vi "CRYDB Create Tables.vi"(8 "error in":errorcluster, 11 "connection reference":T1) -> (0 "error out":errorcluster, 3 "connection reference out":T1)   [LabVIEW 2013]
uses:
  <vilib>/addons/database/Connection.llb/Conn ObjectReference.ctl
  <vilib>/addons/database/Auxilliary.llb/DB Tools Column Info.ctl
  <vilib>/addons/database/Auxilliary.llb/DB Tools DataTypes.ctl
  <vilib>/addons/database/NI_Database_API.lvlib
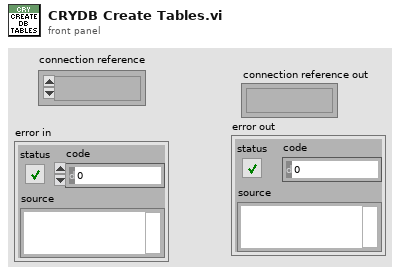
[diagram p1: front panel]
types:
  T1 = typedef "NI_Database_API.lvlib/Conn ObjectReference.ctl" = refnum<k1>
  T2 = typedef "NI_Database_API.lvlib/DB Tools Column Info.ctl" = cluster{"column name":string, "data type":T3, "size":i32, "allow null?":bool}
  T3 = typedef "NI_Database_API.lvlib/DB Tools DataTypes.ctl" = enum16{"String", "Long (I32)", "Single (SGL)", "Double (DBL)", "Date/Time", "Binary"}
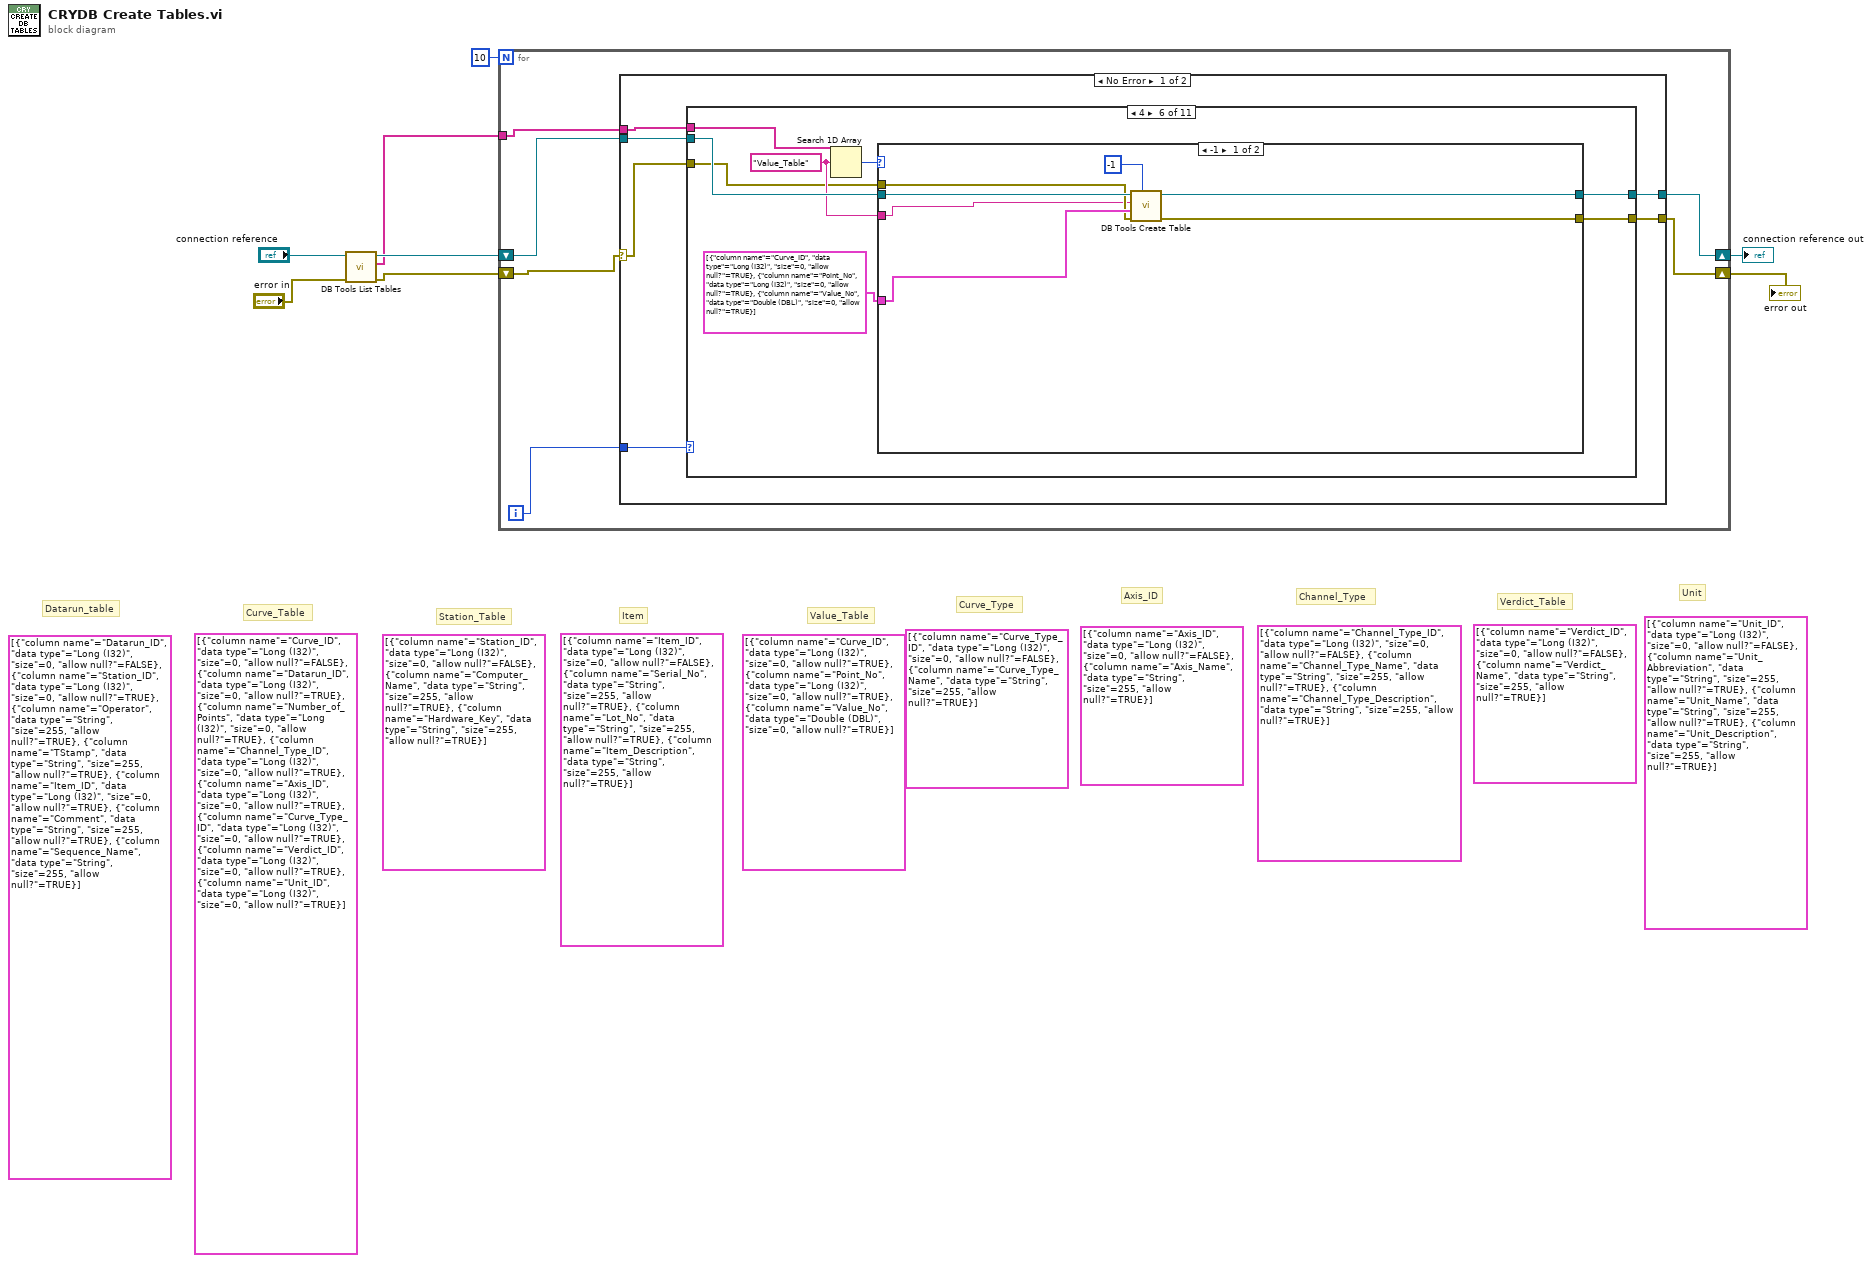
[diagram p0: block diagram]
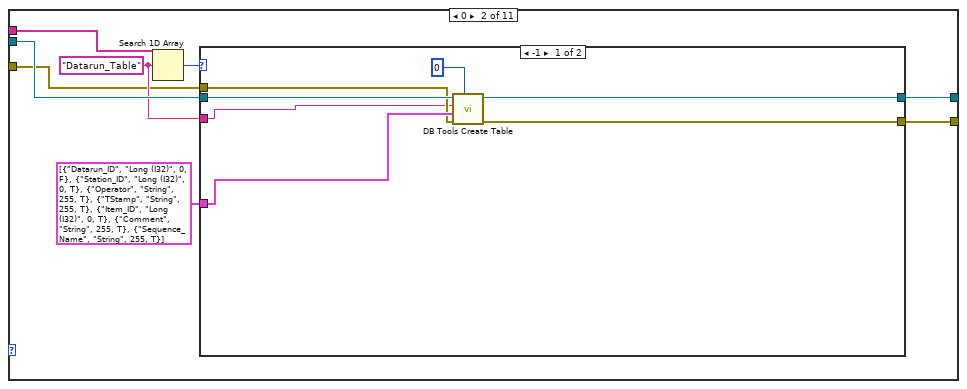
[diagram p3: hidden frame]
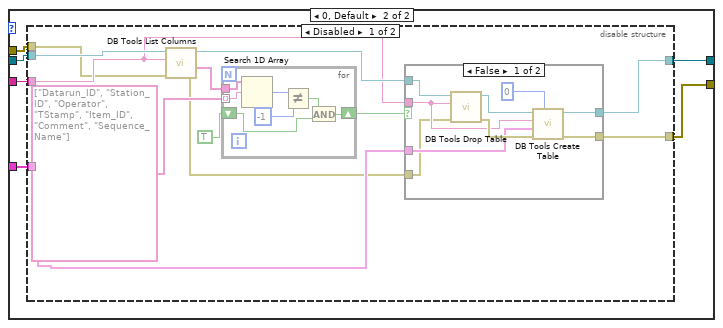
[diagram p4: hidden frame]
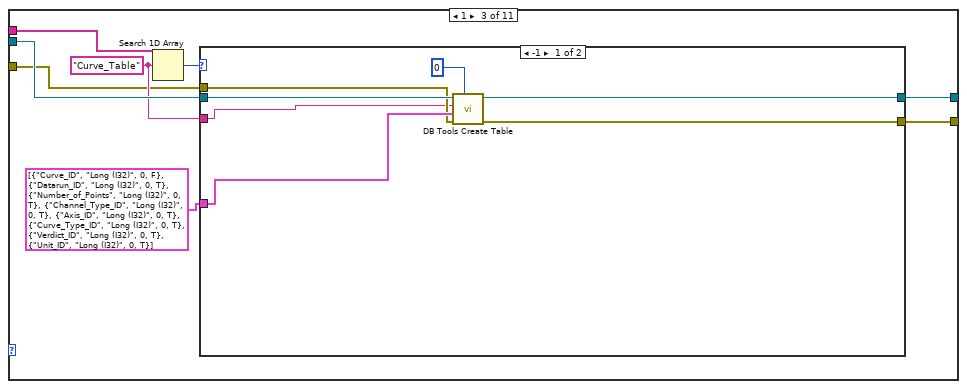
[diagram p7: hidden frame]
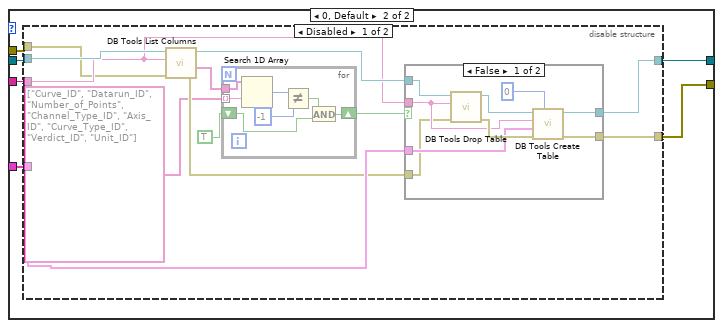
[diagram p8: hidden frame]
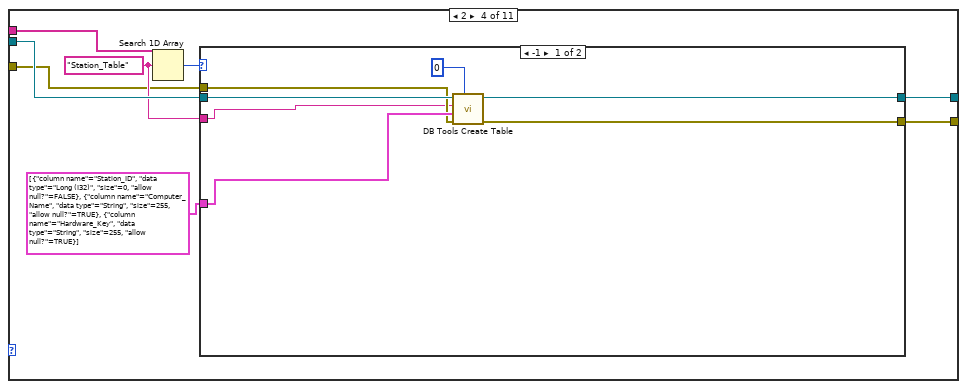
[diagram p11: hidden frame]
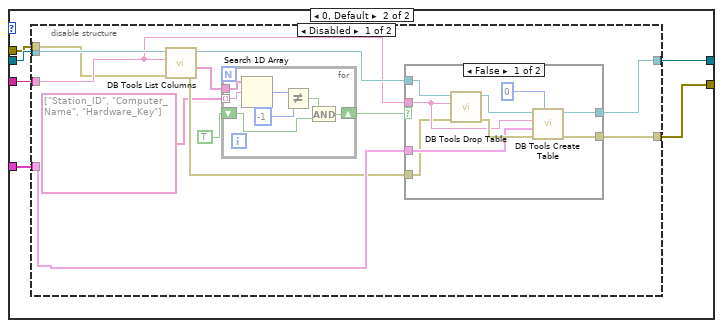
[diagram p12: hidden frame]
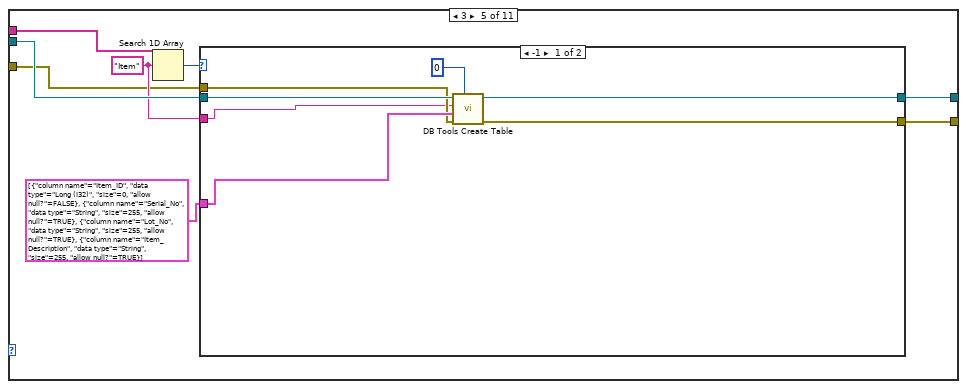
[diagram p15: hidden frame]
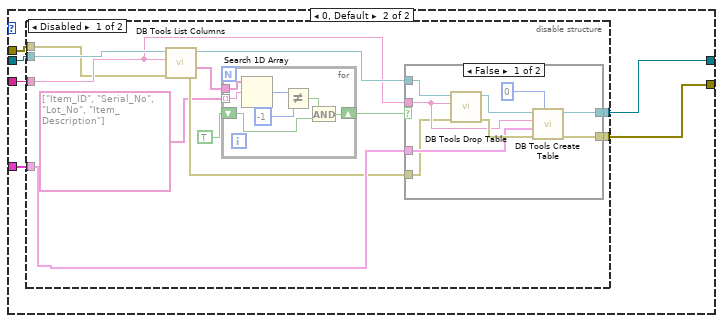
[diagram p16: hidden frame]
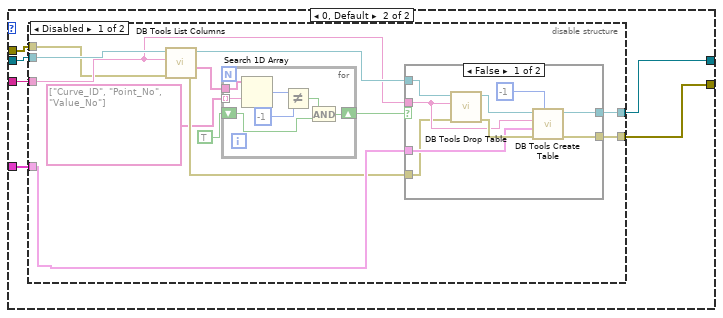
[diagram p19: hidden frame]
diagram:
  (unwired) T2[] [{"column name"="Unit_ID", "data type"=enum."Long (I32)", "size"=0, "allow null?"=FALSE}, {"column name"="Unit_Abbreviation", "data type"=enum."String", "size"=255, "allow null?"=TRUE}, {"column name"="Unit_Name", "data type"=enum."String", "size"=255, "allow null?"=TRUE}, {"column name"="Unit_Description", "data type"=enum."String", "size"=255, "allow null?"=TRUE}] ("column information")
  (unwired) T2[] [{"column name"="Verdict_ID", "data type"=enum."Long (I32)", "size"=0, "allow null?"=FALSE}, {"column name"="Verdict_Name", "data type"=enum."String", "size"=255, "allow null?"=TRUE}] ("column information")
  (unwired) T2[] [{"column name"="Channel_Type_ID", "data type"=enum."Long (I32)", "size"=0, "allow null?"=FALSE}, {"column name"="Channel_Type_Name", "data type"=enum."String", "size"=255, "allow null?"=TRUE}, {"column name"="Channel_Type_Description", "data type"=enum."String", "size"=255, "allow null?"=TRUE}] ("column information")
  (unwired) T2[] [{"column name"="Axis_ID", "data type"=enum."Long (I32)", "size"=0, "allow null?"=FALSE}, {"column name"="Axis_Name", "data type"=enum."String", "size"=255, "allow null?"=TRUE}] ("column information")
  (unwired) T2[] [{"column name"="Curve_Type_ID", "data type"=enum."Long (I32)", "size"=0, "allow null?"=FALSE}, {"column name"="Curve_Type_Name", "data type"=enum."String", "size"=255, "allow null?"=TRUE}] ("column information")
  (unwired) T2[] [{"column name"="Curve_ID", "data type"=enum."Long (I32)", "size"=0, "allow null?"=TRUE}, {"column name"="Point_No", "data type"=enum."Long (I32)", "size"=0, "allow null?"=TRUE}, {"column name"="Value_No", "data type"=enum."Double (DBL)", "size"=0, "allow null?"=TRUE}] ("column information")
  (unwired) T2[] [{"column name"="Item_ID", "data type"=enum."Long (I32)", "size"=0, "allow null?"=FALSE}, {"column name"="Serial_No", "data type"=enum."String", "size"=255, "allow null?"=TRUE}, {"column name"="Lot_No", "data type"=enum."String", "size"=255, "allow null?"=TRUE}, {"column name"="Item_Description", "data type"=enum."String", "size"=255, "allow null?"=TRUE}] ("column information")
  (unwired) T2[] [{"column name"="Station_ID", "data type"=enum."Long (I32)", "size"=0, "allow null?"=FALSE}, {"column name"="Computer_Name", "data type"=enum."String", "size"=255, "allow null?"=TRUE}, {"column name"="Hardware_Key", "data type"=enum."String", "size"=255, "allow null?"=TRUE}] ("column information")
  (unwired) T2[] [{"column name"="Curve_ID", "data type"=enum."Long (I32)", "size"=0, "allow null?"=FALSE}, {"column name"="Datarun_ID", "data type"=enum."Long (I32)", "size"=0, "allow null?"=TRUE}, {"column name"="Number_of_Points", "data type"=enum."Long (I32)", "size"=0, "allow null?"=TRUE}, {"column name"="Channel_Type_ID", "data type"=enum."Long (I32)", "size"=0, "allow null?"=TRUE}, {"column name"="Axis_ID", "data type"=enum."Long (I32)", "size"=0, "allow null?"=TRUE}, {"column name"="Curve_Type_ID", "data type"=enum."Long (I32)", "size"=0, "allow null?"=TRUE}, {"column name"="Verdict_ID", "data type"=enum."Long (I32)", "size"=0, "allow null?"=TRUE}, {"column name"="Unit_ID", "data type"=enum."Long (I32)", "size"=0, "allow null?"=TRUE}] ("column information")
  (unwired) T2[] [{"column name"="Datarun_ID", "data type"=enum."Long (I32)", "size"=0, "allow null?"=FALSE}, {"column name"="Station_ID", "data type"=enum."Long (I32)", "size"=0, "allow null?"=TRUE}, {"column name"="Operator", "data type"=enum."String", "size"=255, "allow null?"=TRUE}, {"column name"="TStamp", "data type"=enum."String", "size"=255, "allow null?"=TRUE}, {"column name"="Item_ID", "data type"=enum."Long (I32)", "size"=0, "allow null?"=TRUE}, {"column name"="Comment", "data type"=enum."String", "size"=255, "allow null?"=TRUE}, {"column name"="Sequence_Name", "data type"=enum."String", "size"=255, "allow null?"=TRUE}] ("column information")
  # "Unit"
  # "Verdict_Table"
  # "Channel_Type"
  # "Axis_ID"
  # "Curve_Type"
  # "Value_Table"
  # "Item"
  # "Station_Table"
  # "Curve_Table"
  # "Datarun_table"
  n1 = call <vilib>:"DB Tools List Tables.vi"("error in (no error)"="error in", "connection reference"="connection reference") -> ("error out"=w2:errorcluster, "tables"=w1:string[], "connection reference out"=w4:T1)  [unwired: 3 in]
  n2 = for {
    N: 10 -> [_]
    shift-right: [w12] -> w7
    shift-left: w4 -> [w14]
    shift-right: [w11] -> w6
    shift-left: w2 -> [w9]
    tunnel: w1 -> [w10]
    i -> [w13]
    n3 = case shown="No Error" w9 {
      selector: w9 -> [w15 w553]
      tunnel: w14 -> [w17 w554]
      tunnel: w13 -> [w20 _]
      tunnel: [w19 w554] -> w12
      tunnel: [w18 w553] -> w11
      tunnel: w10 -> [w16 _]
      frame No Error {
        n4 = case shown="4" w20 {
          tunnel: w16 -> [_ w30 w83 w136 w189 w242 w295 w348 w401 w454 w507]
          tunnel: w17 -> [w22 w29 w82 w135 w188 w241 w294 w347 w400 w453 w506]
          tunnel: [w22 w25 w79 w132 w185 w238 w291 w344 w397 w450 w503] -> w19
          tunnel: [w21 w24 w78 w131 w184 w237 w290 w343 w396 w449 w502] -> w18
          tunnel: w15 -> [w21 w23 w77 w130 w183 w236 w289 w342 w395 w448 w501]
          frame Default {
          }
          frame 0 {
            w27 = "Datarun_Table" ("element")
            n5 = Search 1D Array(1D array=w30, element=w27) -> (index of element=w28:i32)  [unwired: 1 in]
            n6 = case shown="-1" w28 {
              tunnel: w29 -> [w37 w43]
              tunnel: [w35 w40] -> w24
              tunnel: w27 -> [w31 w42]
              tunnel: T2[] [{"column name"="Datarun_ID", "data type"=enum."Long (I32)", "size"=0, "allow null?"=FALSE}, {"column name"="Station_ID", "data type"=enum."Long (I32)", "size"=0, "allow null?"=TRUE}, {"column name"="Operator", "data type"=enum."String", "size"=255, "allow null?"=TRUE}, {"column name"="TStamp", "data type"=enum."String", "size"=255, "allow null?"=TRUE}, {"column name"="Item_ID", "data type"=enum."Long (I32)", "size"=0, "allow null?"=TRUE}, {"column name"="Comment", "data type"=enum."String", "size"=255, "allow null?"=TRUE}, {"column name"="Sequence_Name", "data type"=enum."String", "size"=255, "allow null?"=TRUE}] ("column information") -> [w34 w41]
              tunnel: [w33 w39] -> w25
              tunnel: w23 -> [w32 w38]
              frame -1 {
                n7 = call <vilib>:"DB Tools Create Table.vi"("primary key (-1)"=0, "error in (no error)"=w32, "column information"=w34, "table"=w31, "connection reference"=w37) -> ("error out"=w35:errorcluster, "connection reference out"=w33:T1)  [unwired: 3 in]
              }
              frame 0, Default {
                n8 = disable-structure shown="Disabled" {
                  disable-tunnel: w43 -> [w55 w74]
                  disable-tunnel: w42 -> [w49 _]
                  disable-tunnel: w41 -> [w48 _]
                  disable-tunnel: [w47 w75] -> w40
                  disable-tunnel: [w46 w74] -> w39
                  disable-tunnel: w38 -> [w45 w75]
                  frame Disabled {
                    n9 = call <vilib>:"DB Tools List Columns.vi"("error in (no error)"=w45, "table"=w49, "connection reference"=w55) -> ("error out"=w44:errorcluster, "columns"=w53:string[], "connection reference out"=w50:T1)  [unwired: 1 in, 1 out]
                    n10 = for {
                      tunnel: string[] ["Datarun_ID", "Station_ID", "Operator", "TStamp", "Item_ID", "Comment", "Sequence_Name"] ("columns") -> [w72] mode=indexing
                      tunnel: w53 -> [w73]
                      shift-right: [w67] -> w51
                      shift-left: TRUE -> [w69]
                      n11 = Search 1D Array(1D array=w73, element=w72) -> (index of element=w71:i32)  [unwired: 1 in]
                      n12 = Not Equal?(x=w71, y=-1) -> (x != y?=w68:bool)
                      n13 = And(x=w68, y=w69) -> (x .and. y?=w67:bool)
                    }
                    n14 = case shown="False" w51 {
                      tunnel: w50 -> [w64 w66]
                      tunnel: w49 -> [w60 _]
                      tunnel: w48 -> [w61 _]
                      tunnel: [w58 w65] -> w47
                      tunnel: [w57 w66] -> w46
                      tunnel: w44 -> [w56 w65]
                      frame False {
                        n15 = call <vilib>:"DB Tools Drop Table.vi"("error in (no error)"=w56, "table"=w60, "connection reference"=w64) -> ("error out"=w62:errorcluster, "connection reference out"=w63:T1)  [unwired: 5 in]
                        n16 = call <vilib>:"DB Tools Create Table.vi"("primary key (-1)"=0, "error in (no error)"=w62, "column information"=w61, "table"=w60, "connection reference"=w63) -> ("error out"=w58:errorcluster, "connection reference out"=w57:T1)  [unwired: 3 in]
                      }
                      frame True {
                      }
                    }
                  }
                  frame Enabled {
                  }
                }
              }
            }
          }
          frame 1 {
            w80 = "Curve_Table" ("element")
            n17 = Search 1D Array(1D array=w83, element=w80) -> (index of element=w81:i32)  [unwired: 1 in]
            n18 = case shown="-1" w81 {
              tunnel: w82 -> [w90 w96]
              tunnel: [w88 w93] -> w78
              tunnel: w80 -> [w84 w95]
              tunnel: T2[] [{"column name"="Curve_ID", "data type"=enum."Long (I32)", "size"=0, "allow null?"=FALSE}, {"column name"="Datarun_ID", "data type"=enum."Long (I32)", "size"=0, "allow null?"=TRUE}, {"column name"="Number_of_Points", "data type"=enum."Long (I32)", "size"=0, "allow null?"=TRUE}, {"column name"="Channel_Type_ID", "data type"=enum."Long (I32)", "size"=0, "allow null?"=TRUE}, {"column name"="Axis_ID", "data type"=enum."Long (I32)", "size"=0, "allow null?"=TRUE}, {"column name"="Curve_Type_ID", "data type"=enum."Long (I32)", "size"=0, "allow null?"=TRUE}, {"column name"="Verdict_ID", "data type"=enum."Long (I32)", "size"=0, "allow null?"=TRUE}, {"column name"="Unit_ID", "data type"=enum."Long (I32)", "size"=0, "allow null?"=TRUE}] ("column information") -> [w87 w94]
              tunnel: [w86 w92] -> w79
              tunnel: w77 -> [w85 w91]
              frame -1 {
                n19 = call <vilib>:"DB Tools Create Table.vi"("primary key (-1)"=0, "error in (no error)"=w85, "column information"=w87, "table"=w84, "connection reference"=w90) -> ("error out"=w88:errorcluster, "connection reference out"=w86:T1)  [unwired: 3 in]
              }
              frame 0, Default {
                n20 = disable-structure shown="Disabled" {
                  disable-tunnel: w96 -> [w108 w128]
                  disable-tunnel: w95 -> [w103 _]
                  disable-tunnel: w94 -> [w102 _]
                  disable-tunnel: [w101 w127] -> w93
                  disable-tunnel: [w100 w128] -> w92
                  disable-tunnel: w91 -> [w99 w127]
                  frame Disabled {
                    n21 = call <vilib>:"DB Tools List Columns.vi"("error in (no error)"=w99, "table"=w103, "connection reference"=w108) -> ("error out"=w98:errorcluster, "columns"=w107:string[], "connection reference out"=w104:T1)  [unwired: 1 in, 1 out]
                    n22 = for {
                      tunnel: [w120] -> _ mode=indexing
                      tunnel: w107 -> [w126]
                      shift-right: [w121] -> w105
                      shift-left: TRUE -> [w123]
                      tunnel: string[] ["Curve_ID", "Datarun_ID", "Number_of_Points", "Channel_Type_ID", "Axis_ID", "Curve_Type_ID", "Verdict_ID", "Unit_ID"] ("columns") -> [w120] mode=indexing
                      n23 = Search 1D Array(1D array=w126, element=w120) -> (index of element=w125:i32)  [unwired: 1 in]
                      n24 = Not Equal?(x=w125, y=-1) -> (x != y?=w122:bool)
                      n25 = And(x=w122, y=w123) -> (x .and. y?=w121:bool)
                    }
                    n26 = case shown="False" w105 {
                      tunnel: w104 -> [w117 w119]
                      tunnel: w103 -> [w113 _]
                      tunnel: w102 -> [w114 _]
                      tunnel: [w111 w118] -> w101
                      tunnel: [w110 w119] -> w100
                      tunnel: w98 -> [w109 w118]
                      frame False {
                        n27 = call <vilib>:"DB Tools Drop Table.vi"("error in (no error)"=w109, "table"=w113, "connection reference"=w117) -> ("error out"=w115:errorcluster, "connection reference out"=w116:T1)  [unwired: 5 in]
                        n28 = call <vilib>:"DB Tools Create Table.vi"("primary key (-1)"=0, "error in (no error)"=w115, "column information"=w114, "table"=w113, "connection reference"=w116) -> ("error out"=w111:errorcluster, "connection reference out"=w110:T1)  [unwired: 3 in]
                      }
                      frame True {
                      }
                    }
                  }
                  frame Enabled {
                  }
                }
              }
            }
          }
          frame 2 {
            w133 = "Station_Table" ("element")
            n29 = Search 1D Array(1D array=w136, element=w133) -> (index of element=w134:i32)  [unwired: 1 in]
            n30 = case shown="-1" w134 {
              tunnel: w135 -> [w143 w149]
              tunnel: [w141 w146] -> w131
              tunnel: w133 -> [w137 w148]
              tunnel: T2[] [{"column name"="Station_ID", "data type"=enum."Long (I32)", "size"=0, "allow null?"=FALSE}, {"column name"="Computer_Name", "data type"=enum."String", "size"=255, "allow null?"=TRUE}, {"column name"="Hardware_Key", "data type"=enum."String", "size"=255, "allow null?"=TRUE}] ("column information") -> [w140 w147]
              tunnel: [w139 w145] -> w132
              tunnel: w130 -> [w138 w144]
              frame -1 {
                n31 = call <vilib>:"DB Tools Create Table.vi"("primary key (-1)"=0, "error in (no error)"=w138, "column information"=w140, "table"=w137, "connection reference"=w143) -> ("error out"=w141:errorcluster, "connection reference out"=w139:T1)  [unwired: 3 in]
              }
              frame 0, Default {
                n32 = disable-structure shown="Disabled" {
                  disable-tunnel: w149 -> [w161 w180]
                  disable-tunnel: w148 -> [w156 _]
                  disable-tunnel: w147 -> [w155 _]
                  disable-tunnel: [w154 w181] -> w146
                  disable-tunnel: [w153 w180] -> w145
                  disable-tunnel: w144 -> [w152 w181]
                  frame Disabled {
                    n33 = call <vilib>:"DB Tools List Columns.vi"("error in (no error)"=w152, "table"=w156, "connection reference"=w161) -> ("error out"=w151:errorcluster, "columns"=w160:string[], "connection reference out"=w157:T1)  [unwired: 1 in, 1 out]
                    n34 = for {
                      tunnel: w160 -> [w179]
                      shift-right: [w174] -> w158
                      shift-left: TRUE -> [w176]
                      tunnel: string[] ["Station_ID", "Computer_Name", "Hardware_Key"] ("columns") -> [w173] mode=indexing
                      n35 = Search 1D Array(1D array=w179, element=w173) -> (index of element=w178:i32)  [unwired: 1 in]
                      n36 = Not Equal?(x=w178, y=-1) -> (x != y?=w175:bool)
                      n37 = And(x=w175, y=w176) -> (x .and. y?=w174:bool)
                    }
                    n38 = case shown="False" w158 {
                      tunnel: w157 -> [w170 w172]
                      tunnel: w156 -> [w166 _]
                      tunnel: w155 -> [w167 _]
                      tunnel: [w164 w171] -> w154
                      tunnel: [w163 w172] -> w153
                      tunnel: w151 -> [w162 w171]
                      frame False {
                        n39 = call <vilib>:"DB Tools Drop Table.vi"("error in (no error)"=w162, "table"=w166, "connection reference"=w170) -> ("error out"=w168:errorcluster, "connection reference out"=w169:T1)  [unwired: 5 in]
                        n40 = call <vilib>:"DB Tools Create Table.vi"("primary key (-1)"=0, "error in (no error)"=w168, "column information"=w167, "table"=w166, "connection reference"=w169) -> ("error out"=w164:errorcluster, "connection reference out"=w163:T1)  [unwired: 3 in]
                      }
                      frame True {
                      }
                    }
                  }
                  frame Enabled {
                  }
                }
              }
            }
          }
          frame 3 {
            w186 = "Item" ("element")
            n41 = Search 1D Array(1D array=w189, element=w186) -> (index of element=w187:i32)  [unwired: 1 in]
            n42 = case shown="-1" w187 {
              tunnel: w188 -> [w196 w202]
              tunnel: [w194 w199] -> w184
              tunnel: w186 -> [w190 w201]
              tunnel: T2[] [{"column name"="Item_ID", "data type"=enum."Long (I32)", "size"=0, "allow null?"=FALSE}, {"column name"="Serial_No", "data type"=enum."String", "size"=255, "allow null?"=TRUE}, {"column name"="Lot_No", "data type"=enum."String", "size"=255, "allow null?"=TRUE}, {"column name"="Item_Description", "data type"=enum."String", "size"=255, "allow null?"=TRUE}] ("column information") -> [w193 w200]
              tunnel: [w192 w198] -> w185
              tunnel: w183 -> [w191 w197]
              frame -1 {
                n43 = call <vilib>:"DB Tools Create Table.vi"("primary key (-1)"=0, "error in (no error)"=w191, "column information"=w193, "table"=w190, "connection reference"=w196) -> ("error out"=w194:errorcluster, "connection reference out"=w192:T1)  [unwired: 3 in]
              }
              frame 0, Default {
                n44 = disable-structure shown="Disabled" {
                  disable-tunnel: w202 -> [w214 w234]
                  disable-tunnel: w201 -> [w209 _]
                  disable-tunnel: w200 -> [w208 _]
                  disable-tunnel: [w207 w233] -> w199
                  disable-tunnel: [w206 w234] -> w198
                  disable-tunnel: w197 -> [w205 w233]
                  frame Disabled {
                    n45 = call <vilib>:"DB Tools List Columns.vi"("error in (no error)"=w205, "table"=w209, "connection reference"=w214) -> ("error out"=w204:errorcluster, "columns"=w213:string[], "connection reference out"=w210:T1)  [unwired: 1 in, 1 out]
                    n46 = for {
                      tunnel: w213 -> [w232]
                      shift-right: [w227] -> w211
                      shift-left: TRUE -> [w229]
                      tunnel: string[] ["Item_ID", "Serial_No", "Lot_No", "Item_Description"] ("columns") -> [w226] mode=indexing
                      n47 = Search 1D Array(1D array=w232, element=w226) -> (index of element=w231:i32)  [unwired: 1 in]
                      n48 = Not Equal?(x=w231, y=-1) -> (x != y?=w228:bool)
                      n49 = And(x=w228, y=w229) -> (x .and. y?=w227:bool)
                    }
                    n50 = case shown="False" w211 {
                      tunnel: w210 -> [w223 w225]
                      tunnel: w209 -> [w219 _]
                      tunnel: w208 -> [w220 _]
                      tunnel: [w217 w224] -> w207
                      tunnel: [w216 w225] -> w206
                      tunnel: w204 -> [w215 w224]
                      frame False {
                        n51 = call <vilib>:"DB Tools Drop Table.vi"("error in (no error)"=w215, "table"=w219, "connection reference"=w223) -> ("error out"=w221:errorcluster, "connection reference out"=w222:T1)  [unwired: 5 in]
                        n52 = call <vilib>:"DB Tools Create Table.vi"("primary key (-1)"=0, "error in (no error)"=w221, "column information"=w220, "table"=w219, "connection reference"=w222) -> ("error out"=w217:errorcluster, "connection reference out"=w216:T1)  [unwired: 3 in]
                      }
                      frame True {
                      }
                    }
                  }
                  frame Enabled {
                  }
                }
              }
            }
          }
          frame 4 {
            w239 = "Value_Table" ("element")
            n53 = Search 1D Array(1D array=w242, element=w239) -> (index of element=w240:i32)  [unwired: 1 in]
            n54 = case shown="-1" w240 {
              tunnel: w241 -> [w249 w255]
              tunnel: [w247 w252] -> w237
              tunnel: w239 -> [w243 w254]
              tunnel: T2[] [{"column name"="Curve_ID", "data type"=enum."Long (I32)", "size"=0, "allow null?"=TRUE}, {"column name"="Point_No", "data type"=enum."Long (I32)", "size"=0, "allow null?"=TRUE}, {"column name"="Value_No", "data type"=enum."Double (DBL)", "size"=0, "allow null?"=TRUE}] ("column information") -> [w246 w253]
              tunnel: [w245 w251] -> w238
              tunnel: w236 -> [w244 w250]
              frame -1 {
                n55 = call <vilib>:"DB Tools Create Table.vi"("primary key (-1)"=-1, "error in (no error)"=w244, "column information"=w246, "table"=w243, "connection reference"=w249) -> ("error out"=w247:errorcluster, "connection reference out"=w245:T1)  [unwired: 3 in]
              }
              frame 0, Default {
                n56 = disable-structure shown="Disabled" {
                  disable-tunnel: w255 -> [w267 w287]
                  disable-tunnel: w254 -> [w262 _]
                  disable-tunnel: w253 -> [w261 _]
                  disable-tunnel: [w260 w286] -> w252
                  disable-tunnel: [w259 w287] -> w251
                  disable-tunnel: w250 -> [w258 w286]
                  frame Disabled {
                    n57 = call <vilib>:"DB Tools List Columns.vi"("error in (no error)"=w258, "table"=w262, "connection reference"=w267) -> ("error out"=w257:errorcluster, "columns"=w266:string[], "connection reference out"=w263:T1)  [unwired: 1 in, 1 out]
                    n58 = for {
                      tunnel: w266 -> [w285]
                      shift-right: [w280] -> w264
                      shift-left: TRUE -> [w282]
                      tunnel: [w279] -> _ mode=indexing
                      tunnel: string[] ["Curve_ID", "Point_No", "Value_No"] ("columns") -> [w279] mode=indexing
                      n59 = Search 1D Array(1D array=w285, element=w279) -> (index of element=w284:i32)  [unwired: 1 in]
                      n60 = Not Equal?(x=w284, y=-1) -> (x != y?=w281:bool)
                      n61 = And(x=w281, y=w282) -> (x .and. y?=w280:bool)
                    }
                    n62 = case shown="False" w264 {
                      tunnel: w263 -> [w276 w278]
                      tunnel: w262 -> [w272 _]
                      tunnel: w261 -> [w273 _]
                      tunnel: [w270 w277] -> w260
                      tunnel: [w269 w278] -> w259
                      tunnel: w257 -> [w268 w277]
                      frame False {
                        n63 = call <vilib>:"DB Tools Drop Table.vi"("error in (no error)"=w268, "table"=w272, "connection reference"=w276) -> ("error out"=w274:errorcluster, "connection reference out"=w275:T1)  [unwired: 5 in]
                        n64 = call <vilib>:"DB Tools Create Table.vi"("primary key (-1)"=-1, "error in (no error)"=w274, "column information"=w273, "table"=w272, "connection reference"=w275) -> ("error out"=w270:errorcluster, "connection reference out"=w269:T1)  [unwired: 3 in]
                      }
                      frame True {
                      }
                    }
                  }
                  frame Enabled {
                  }
                }
              }
            }
          }
          frame 5 {
            w292 = "Curve_Type" ("element")
            n65 = Search 1D Array(1D array=w295, element=w292) -> (index of element=w293:i32)  [unwired: 1 in]
            n66 = case shown="-1" w293 {
              tunnel: w294 -> [w302 w308]
              tunnel: [w300 w305] -> w290
              tunnel: w292 -> [w296 w307]
              tunnel: T2[] [{"column name"="Curve_Type_ID", "data type"=enum."Long (I32)", "size"=0, "allow null?"=FALSE}, {"column name"="Curve_Type_Name", "data type"=enum."String", "size"=255, "allow null?"=TRUE}] ("column information") -> [w299 w306]
              tunnel: [w298 w304] -> w291
              tunnel: w289 -> [w297 w303]
              frame -1 {
                n67 = call <vilib>:"DB Tools Create Table.vi"("primary key (-1)"=0, "error in (no error)"=w297, "column information"=w299, "table"=w296, "connection reference"=w302) -> ("error out"=w300:errorcluster, "connection reference out"=w298:T1)  [unwired: 3 in]
              }
              frame 0, Default {
                n68 = disable-structure shown="Disabled" {
                  disable-tunnel: w308 -> [w320 w339]
                  disable-tunnel: w307 -> [w315 _]
                  disable-tunnel: w306 -> [w314 _]
                  disable-tunnel: [w313 w340] -> w305
                  disable-tunnel: [w312 w339] -> w304
                  disable-tunnel: w303 -> [w311 w340]
                  frame Disabled {
                    n69 = call <vilib>:"DB Tools List Columns.vi"("error in (no error)"=w311, "table"=w315, "connection reference"=w320) -> ("error out"=w310:errorcluster, "columns"=w319:string[], "connection reference out"=w316:T1)  [unwired: 1 in, 1 out]
                    n70 = for {
                      tunnel: w319 -> [w338]
                      shift-right: [w333] -> w317
                      shift-left: TRUE -> [w335]
                      tunnel: [w332] -> _ mode=indexing
                      tunnel: string[] ["Curve_Type_ID", "Curve_Type_Name"] ("columns") -> [w332] mode=indexing
                      n71 = Search 1D Array(1D array=w338, element=w332) -> (index of element=w337:i32)  [unwired: 1 in]
                      n72 = Not Equal?(x=w337, y=-1) -> (x != y?=w334:bool)
                      n73 = And(x=w334, y=w335) -> (x .and. y?=w333:bool)
                    }
                    n74 = case shown="False" w317 {
                      tunnel: w316 -> [w329 w331]
                      tunnel: w315 -> [w325 _]
                      tunnel: w314 -> [w326 _]
                      tunnel: [w323 w330] -> w313
                      tunnel: [w322 w331] -> w312
                      tunnel: w310 -> [w321 w330]
                      frame False {
                        n75 = call <vilib>:"DB Tools Drop Table.vi"("error in (no error)"=w321, "table"=w325, "connection reference"=w329) -> ("error out"=w327:errorcluster, "connection reference out"=w328:T1)  [unwired: 5 in]
                        n76 = call <vilib>:"DB Tools Create Table.vi"("primary key (-1)"=0, "error in (no error)"=w327, "column information"=w326, "table"=w325, "connection reference"=w328) -> ("error out"=w323:errorcluster, "connection reference out"=w322:T1)  [unwired: 3 in]
                      }
                      frame True {
                      }
                    }
                  }
                  frame Enabled {
                  }
                }
              }
            }
          }
          frame 6 {
            w345 = "Axis_ID" ("element")
            n77 = Search 1D Array(1D array=w348, element=w345) -> (index of element=w346:i32)  [unwired: 1 in]
            n78 = case shown="-1" w346 {
              tunnel: w347 -> [w355 w361]
              tunnel: [w353 w358] -> w343
              tunnel: w345 -> [w349 w360]
              tunnel: T2[] [{"column name"="Axis_ID", "data type"=enum."Long (I32)", "size"=0, "allow null?"=FALSE}, {"column name"="Axis_Name", "data type"=enum."String", "size"=255, "allow null?"=TRUE}] ("column information") -> [w352 w359]
              tunnel: [w351 w357] -> w344
              tunnel: w342 -> [w350 w356]
              frame -1 {
                n79 = call <vilib>:"DB Tools Create Table.vi"("primary key (-1)"=0, "error in (no error)"=w350, "column information"=w352, "table"=w349, "connection reference"=w355) -> ("error out"=w353:errorcluster, "connection reference out"=w351:T1)  [unwired: 3 in]
              }
              frame 0, Default {
                n80 = disable-structure shown="Disabled" {
                  disable-tunnel: w361 -> [w373 w393]
                  disable-tunnel: w360 -> [w368 _]
                  disable-tunnel: w359 -> [w367 _]
                  disable-tunnel: [w366 w392] -> w358
                  disable-tunnel: [w365 w393] -> w357
                  disable-tunnel: w356 -> [w364 w392]
                  frame Disabled {
                    n81 = call <vilib>:"DB Tools List Columns.vi"("error in (no error)"=w364, "table"=w368, "connection reference"=w373) -> ("error out"=w363:errorcluster, "columns"=w372:string[], "connection reference out"=w369:T1)  [unwired: 1 in, 1 out]
                    n82 = for {
                      tunnel: w372 -> [w391]
                      shift-right: [w386] -> w370
                      shift-left: TRUE -> [w388]
                      tunnel: [w385] -> _ mode=indexing
                      tunnel: string[] ["Axis_ID", "Axis_Name"] ("columns") -> [w385] mode=indexing
                      n83 = Search 1D Array(1D array=w391, element=w385) -> (index of element=w390:i32)  [unwired: 1 in]
                      n84 = Not Equal?(x=w390, y=-1) -> (x != y?=w387:bool)
                      n85 = And(x=w387, y=w388) -> (x .and. y?=w386:bool)
                    }
                    n86 = case shown="False" w370 {
                      tunnel: w369 -> [w382 w384]
                      tunnel: w368 -> [w378 _]
                      tunnel: w367 -> [w379 _]
                      tunnel: [w376 w383] -> w366
                      tunnel: [w375 w384] -> w365
                      tunnel: w363 -> [w374 w383]
                      frame False {
                        n87 = call <vilib>:"DB Tools Drop Table.vi"("error in (no error)"=w374, "table"=w378, "connection reference"=w382) -> ("error out"=w380:errorcluster, "connection reference out"=w381:T1)  [unwired: 5 in]
                        n88 = call <vilib>:"DB Tools Create Table.vi"("primary key (-1)"=0, "error in (no error)"=w380, "column information"=w379, "table"=w378, "connection reference"=w381) -> ("error out"=w376:errorcluster, "connection reference out"=w375:T1)  [unwired: 3 in]
                      }
                      frame True {
                      }
                    }
                  }
                  frame Enabled {
                  }
                }
              }
            }
          }
          frame 7 {
            w398 = "Channel_Type" ("element")
            n89 = Search 1D Array(1D array=w401, element=w398) -> (index of element=w399:i32)  [unwired: 1 in]
            n90 = case shown="-1" w399 {
              tunnel: w400 -> [w408 w414]
              tunnel: [w406 w411] -> w396
              tunnel: w398 -> [w402 w413]
              tunnel: T2[] [{"column name"="Channel_Type_ID", "data type"=enum."Long (I32)", "size"=0, "allow null?"=FALSE}, {"column name"="Channel_Type_Name", "data type"=enum."String", "size"=255, "allow null?"=TRUE}, {"column name"="Channel_Type_Description", "data type"=enum."String", "size"=255, "allow null?"=TRUE}] ("column information") -> [w405 w412]
              tunnel: [w404 w410] -> w397
              tunnel: w395 -> [w403 w409]
              frame -1 {
                n91 = call <vilib>:"DB Tools Create Table.vi"("primary key (-1)"=0, "error in (no error)"=w403, "column information"=w405, "table"=w402, "connection reference"=w408) -> ("error out"=w406:errorcluster, "connection reference out"=w404:T1)  [unwired: 3 in]
              }
              frame 0, Default {
                n92 = disable-structure shown="Disabled" {
                  disable-tunnel: w414 -> [w426 w445]
                  disable-tunnel: w413 -> [w421 _]
                  disable-tunnel: w412 -> [w420 _]
                  disable-tunnel: [w419 w446] -> w411
                  disable-tunnel: [w418 w445] -> w410
                  disable-tunnel: w409 -> [w417 w446]
                  frame Disabled {
                    n93 = call <vilib>:"DB Tools List Columns.vi"("error in (no error)"=w417, "table"=w421, "connection reference"=w426) -> ("error out"=w416:errorcluster, "columns"=w425:string[], "connection reference out"=w422:T1)  [unwired: 1 in, 1 out]
                    n94 = for {
                      tunnel: w425 -> [w444]
                      shift-right: [w439] -> w423
                      shift-left: TRUE -> [w441]
                      tunnel: [w438] -> _ mode=indexing
                      tunnel: string[] ["Channel_Type_ID", "Channel_Type_Name", "Channel_Type_Description"] ("columns") -> [w438] mode=indexing
                      n95 = Search 1D Array(1D array=w444, element=w438) -> (index of element=w443:i32)  [unwired: 1 in]
                      n96 = Not Equal?(x=w443, y=-1) -> (x != y?=w440:bool)
                      n97 = And(x=w440, y=w441) -> (x .and. y?=w439:bool)
                    }
                    n98 = case shown="False" w423 {
                      tunnel: w422 -> [w435 w437]
                      tunnel: w421 -> [w431 _]
                      tunnel: w420 -> [w432 _]
                      tunnel: [w429 w436] -> w419
                      tunnel: [w428 w437] -> w418
                      tunnel: w416 -> [w427 w436]
                      frame False {
                        n99 = call <vilib>:"DB Tools Drop Table.vi"("error in (no error)"=w427, "table"=w431, "connection reference"=w435) -> ("error out"=w433:errorcluster, "connection reference out"=w434:T1)  [unwired: 5 in]
                        n100 = call <vilib>:"DB Tools Create Table.vi"("primary key (-1)"=0, "error in (no error)"=w433, "column information"=w432, "table"=w431, "connection reference"=w434) -> ("error out"=w429:errorcluster, "connection reference out"=w428:T1)  [unwired: 3 in]
                      }
                      frame True {
                      }
                    }
                  }
                  frame Enabled {
                  }
                }
              }
            }
          }
          frame 8 {
            w451 = "Verdict_Table" ("element")
            n101 = Search 1D Array(1D array=w454, element=w451) -> (index of element=w452:i32)  [unwired: 1 in]
            n102 = case shown="-1" w452 {
              tunnel: w453 -> [w461 w467]
              tunnel: [w459 w464] -> w449
              tunnel: w451 -> [w455 w466]
              tunnel: T2[] [{"column name"="Verdict_ID", "data type"=enum."Long (I32)", "size"=0, "allow null?"=FALSE}, {"column name"="Verdict_Name", "data type"=enum."String", "size"=255, "allow null?"=TRUE}] ("column information") -> [w458 w465]
              tunnel: [w457 w463] -> w450
              tunnel: w448 -> [w456 w462]
              frame -1 {
                n103 = call <vilib>:"DB Tools Create Table.vi"("primary key (-1)"=0, "error in (no error)"=w456, "column information"=w458, "table"=w455, "connection reference"=w461) -> ("error out"=w459:errorcluster, "connection reference out"=w457:T1)  [unwired: 3 in]
              }
              frame 0, Default {
                n104 = disable-structure shown="Disabled" {
                  disable-tunnel: w467 -> [w479 w498]
                  disable-tunnel: w466 -> [w474 _]
                  disable-tunnel: w465 -> [w473 _]
                  disable-tunnel: [w472 w499] -> w464
                  disable-tunnel: [w471 w498] -> w463
                  disable-tunnel: w462 -> [w470 w499]
                  frame Disabled {
                    n105 = call <vilib>:"DB Tools List Columns.vi"("error in (no error)"=w470, "table"=w474, "connection reference"=w479) -> ("error out"=w469:errorcluster, "columns"=w478:string[], "connection reference out"=w475:T1)  [unwired: 1 in, 1 out]
                    n106 = for {
                      tunnel: w478 -> [w497]
                      shift-right: [w492] -> w476
                      shift-left: TRUE -> [w494]
                      tunnel: string[] ["Verdict_ID", "Verdict_Name"] ("columns") -> [w491] mode=indexing
                      n107 = Search 1D Array(1D array=w497, element=w491) -> (index of element=w496:i32)  [unwired: 1 in]
                      n108 = Not Equal?(x=w496, y=-1) -> (x != y?=w493:bool)
                      n109 = And(x=w493, y=w494) -> (x .and. y?=w492:bool)
                    }
                    n110 = case shown="False" w476 {
                      tunnel: w475 -> [w488 w490]
                      tunnel: w474 -> [w484 _]
                      tunnel: w473 -> [w485 _]
                      tunnel: [w482 w489] -> w472
                      tunnel: [w481 w490] -> w471
                      tunnel: w469 -> [w480 w489]
                      frame False {
                        n111 = call <vilib>:"DB Tools Drop Table.vi"("error in (no error)"=w480, "table"=w484, "connection reference"=w488) -> ("error out"=w486:errorcluster, "connection reference out"=w487:T1)  [unwired: 5 in]
                        n112 = call <vilib>:"DB Tools Create Table.vi"("primary key (-1)"=0, "error in (no error)"=w486, "column information"=w485, "table"=w484, "connection reference"=w487) -> ("error out"=w482:errorcluster, "connection reference out"=w481:T1)  [unwired: 3 in]
                      }
                      frame True {
                      }
                    }
                  }
                  frame Enabled {
                  }
                }
              }
            }
          }
          frame 9 {
            w504 = "Unit" ("element")
            n113 = Search 1D Array(1D array=w507, element=w504) -> (index of element=w505:i32)  [unwired: 1 in]
            n114 = case shown="-1" w505 {
              tunnel: w506 -> [w514 w520]
              tunnel: [w512 w517] -> w502
              tunnel: w504 -> [w508 w519]
              tunnel: T2[] [{"column name"="Unit_ID", "data type"=enum."Long (I32)", "size"=0, "allow null?"=FALSE}, {"column name"="Unit_Abbreviation", "data type"=enum."String", "size"=255, "allow null?"=TRUE}, {"column name"="Unit_Name", "data type"=enum."String", "size"=255, "allow null?"=TRUE}, {"column name"="Unit_Description", "data type"=enum."String", "size"=255, "allow null?"=TRUE}] ("column information") -> [w511 w518]
              tunnel: [w510 w516] -> w503
              tunnel: w501 -> [w509 w515]
              frame -1 {
                n115 = call <vilib>:"DB Tools Create Table.vi"("primary key (-1)"=0, "error in (no error)"=w509, "column information"=w511, "table"=w508, "connection reference"=w514) -> ("error out"=w512:errorcluster, "connection reference out"=w510:T1)  [unwired: 3 in]
              }
              frame 0, Default {
                n116 = disable-structure shown="Disabled" {
                  disable-tunnel: w520 -> [w532 w551]
                  disable-tunnel: w519 -> [w527 _]
                  disable-tunnel: w518 -> [w526 _]
                  disable-tunnel: [w525 w552] -> w517
                  disable-tunnel: [w524 w551] -> w516
                  disable-tunnel: w515 -> [w523 w552]
                  frame Disabled {
                    n117 = call <vilib>:"DB Tools List Columns.vi"("error in (no error)"=w523, "table"=w527, "connection reference"=w532) -> ("error out"=w522:errorcluster, "columns"=w531:string[], "connection reference out"=w528:T1)  [unwired: 1 in, 1 out]
                    n118 = for {
                      tunnel: w531 -> [w550]
                      shift-right: [w545] -> w529
                      shift-left: TRUE -> [w547]
                      tunnel: string[] ["Unit_ID", "Unit_Abbreviation", "Unit_Name", "Unit_Description"] ("columns") -> [w544] mode=indexing
                      n119 = Search 1D Array(1D array=w550, element=w544) -> (index of element=w549:i32)  [unwired: 1 in]
                      n120 = Not Equal?(x=w549, y=-1) -> (x != y?=w546:bool)
                      n121 = And(x=w546, y=w547) -> (x .and. y?=w545:bool)
                    }
                    n122 = case shown="False" w529 {
                      tunnel: w528 -> [w541 w543]
                      tunnel: w527 -> [w537 _]
                      tunnel: w526 -> [w538 _]
                      tunnel: [w535 w542] -> w525
                      tunnel: [w534 w543] -> w524
                      tunnel: w522 -> [w533 w542]
                      frame False {
                        n123 = call <vilib>:"DB Tools Drop Table.vi"("error in (no error)"=w533, "table"=w537, "connection reference"=w541) -> ("error out"=w539:errorcluster, "connection reference out"=w540:T1)  [unwired: 5 in]
                        n124 = call <vilib>:"DB Tools Create Table.vi"("primary key (-1)"=0, "error in (no error)"=w539, "column information"=w538, "table"=w537, "connection reference"=w540) -> ("error out"=w535:errorcluster, "connection reference out"=w534:T1)  [unwired: 3 in]
                      }
                      frame True {
                      }
                    }
                  }
                  frame Enabled {
                  }
                }
              }
            }
          }
        }
      }
      frame Error {
      }
    }
  }
  "connection reference out" <- w7
  "error out" <- w6
